vi "Login.vi"(8 "error in (no error)":errorcluster) -> (0 "error out":errorcluster, 2 "Login Successed":bool, 3 "UserName":string)   [LabVIEW 2018]
doc: "Login Form\n\nGet user data from Logins.txt. It is a .iniconfiguration file with Login section where each item has the form:\nUserId=Password,USerName"
uses:
  <vilib>/Utility/error.llb/Error Cluster From Error Code.vi
  <vilib>/ErrorRing/Error Ring.xnode
panel:
  out "Color Box":u32(colorbox)
  out "list of Users":string
  in  "UserID":string
  in  "Password":string
  in  "stop":bool
  in  "Login":bool
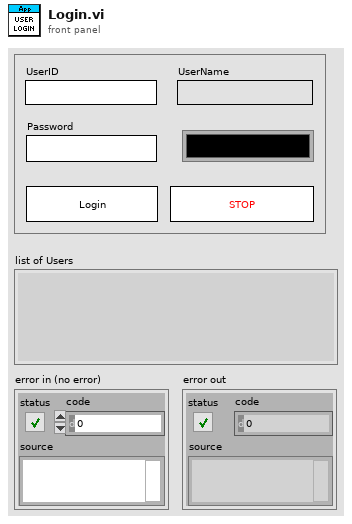
[diagram p1: front panel]
types:
  T1 = enum32{"Invalid", "Standard", "Closed", "Hidden", "Minimized", "Maximized"}
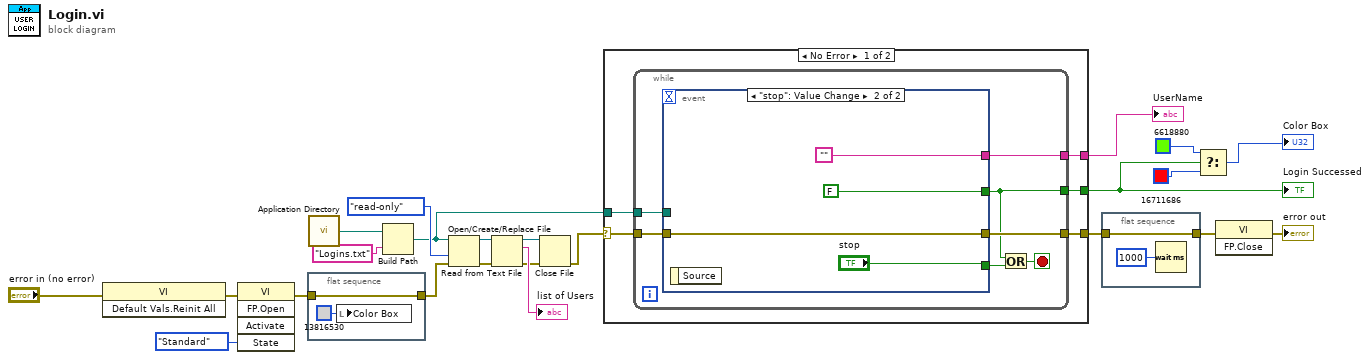
[diagram p0: block diagram]
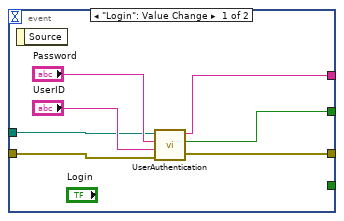
[diagram p2: hidden frame]
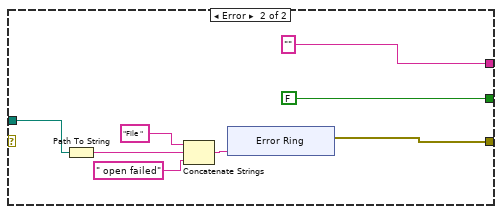
[diagram p3: hidden frame]
diagram:
  n1 = invoke class="VI" method="Default Vals.Reinit All"(error in="error in (no error)") -> (error out=w14:errorcluster)  [unwired: 2 in, 2 out]
  n2 = invoke class="VI" method="FP.Open"(error in=w14, "State"=T1."Standard") -> (error out=w3:errorcluster)  [unwired: 3 in, 4 out]
  n3 = flat-sequence {
    tunnel: [w24] -> w4
    tunnel: w3 -> [w24]
    frame #0 {
      n4 = local write "Color Box"(u32 13816530 ("Color Box")) -> ()
    }
  }
  n5 = call <vilib>:"Application Directory.vi"() -> ("Application Directory"=w1:path)
  n6 = Build Path(base path=w1, name or relative path="Logins.txt") -> (appended path=w5:path)
  n7 = Open/Create/Replace File(file path (use dialog)=w5, error in=w4, access (0:read/write)=enum16{"read/write", "read-only", "write-only"}."read-only") -> (refnum out=w18:refnum<file>, error out=w19:errorcluster)  [unwired: 3 in, 1 out]
  n8 = Read from Text File(file (use dialog)=w18, error in=w19) -> (refnum out=w17:refnum<file>, text=→"list of Users":string, error out=w16:errorcluster)  [unwired: 2 in, 1 out]
  n9 = Close File(refnum=w17, error in=w16) -> (error out=w15:errorcluster)  [unwired: 1 out]
  n10 = case shown="No Error" w15 {
    selector: w15 -> [w26 _]
    tunnel: w5 -> [w30 w55]
    tunnel: [w28 "" ("value")] -> w21
    tunnel: [w27 FALSE ("Visible")] -> w9
    tunnel: [w29 w49] -> w11
    frame No Error {
      n11 = while {
        tunnel: w30 -> [w37]
        tunnel: [w34] -> w29
        tunnel: [w33] -> w28
        tunnel: [w32] -> w27
        tunnel: w26 -> [w31]
        stop <- w35 stop-if-true
        n12 = event shown="[1] \"stop\": Value Change" {
          selector: _ -> [_ _]
          dyn-events: _ -> [_ _]
          timeout: _ -> [_ _]
          tunnel: [w44 w45] -> w34
          tunnel: [_ "stop"] -> w36
          tunnel: w37 -> [w41 _]
          tunnel: [w40 ""] -> w33
          tunnel: w31 -> [w39 w45]
          tunnel: [w38 FALSE ("Boolean")] -> w32
          event "Login": Value Change {
            n13 = event-data() -> ()  [unwired: 1 in, 1 out]
            n14 = call "UserAuthentication.vi"("error in (no error)"=w39, "UserID"="UserID", "Password"="Password", "path"=w41) -> ("error out"=w44:errorcluster, "Boolean"=w38:bool, "UserName"=w40:string)  [unwired: 5 in]
          }
          event "stop": Value Change {
            n15 = event-data() -> ()  [unwired: 1 in, 1 out]
          }
        }
        n16 = Or(x=w32, y=w36) -> (x .or. y?=w35:bool)
      }
    }
    frame Error {
      n17 = Path To String(path=w55) -> (string=w53:string)
      n18 = Concatenate Strings("File " ("string"), w53, " open failed" ("string")) -> (w50:string)
      n19 = xnode "Error Ring"("parameter 0"=w50) -> ("error out"=w49:errorcluster)
    }
  }
  "UserName" <- w21
  "Login Successed" <- w9
  n20 = flat-sequence {
    tunnel: w11 -> [w65]
    tunnel: [w65] -> w10
    frame #0 {
      n21 = Wait (ms)(milliseconds to wait=u32 1000) -> ()  [unwired: 1 out]
    }
  }
  n22 = Select(t=u32 6618880 ("Color Box"), s=w9, f=u32 16711686 ("Color Box")) -> (s? t:f=→"Color Box":u32)
  n23 = invoke class="VI" method="FP.Close"(error in=w10) -> (error out=→"error out":errorcluster)  [unwired: 2 in, 2 out]
